vi "read_params.vi"(8 "error in (no error)":errorcluster, 11 "RidgeCV in":refnum<class "RidgeCV.lvclass">) -> (0 "error out":errorcluster, 2 "params":T1={"alphas"=[0.1, 1.0, 10.0], "fit_intercept"=TRUE, "normalize"=FALSE, "scoring"="None", "cv"=5.0, "gcv_mode"="auto", "store_cv_values"=FALSE, "alpha_per_target"=FALSE}, 3 "RidgeCV out":refnum<class "RidgeCV.lvclass">)   [LabVIEW 2020, in "RidgeCV.lvclass"]
uses:
  RidgeCV.lvclass
  Controls/ridge_cv_params.ctl
  RidgeCV.lvclass/RidgeCV.ctl
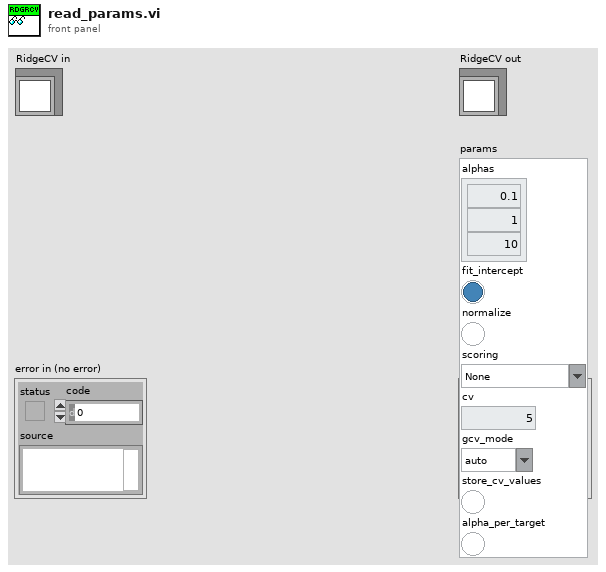
[diagram p1: front panel]
types:
  T1 = typedef "ridge_cv_params.ctl" = cluster{"alphas":dbl[], "fit_intercept":bool, "normalize":bool, "scoring":string, "cv":dbl, "gcv_mode":string, "store_cv_values":bool, "alpha_per_target":bool}
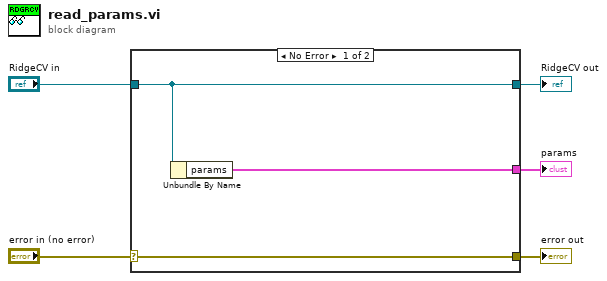
[diagram p0: block diagram]
diagram:
  n1 = case shown="No Error" "error in (no error)" {
    selector: "error in (no error)" -> [w8 w9]
    tunnel: [w8 w9] -> w4
    tunnel: [w7 w10] -> w2
    tunnel: "RidgeCV in" -> [w7 w10]
    tunnel: [w6 _] -> w1
    frame No Error {
      n2 = Unbundle By Name(w7) -> ("params"=w6:T1)
    }
    frame Error {
    }
  }
  "error out" <- w4
  "RidgeCV out" <- w2
  "params" <- w1
